vi "AddRealMeasure.vi"(6 "MeasureExecutionStatus (NOT_COMPLETED)":T1=enum."NOT_COMPLETED", 7 "MeasureTime (Now)":timestamp, 8 "error in":errorcluster, 9 "Precision (6)":u8=6, 10 "Value":dbl, 11 "StepRun in":refnum<class "StepRun.lvclass">) -> (0 "error out":errorcluster, 2 "RealMeasure":refnum<class "RealMeasure.lvclass">, 3 "StepRun out":refnum<class "StepRun.lvclass">)   [LabVIEW 2021, in "ProligentXMLGenerator.lvlib" / "StepRun.lvclass"]
doc: "Add a Measure.\n\nDefines the value acquired by the measure.\nMeasures are globaly unique by their MeasureId property."
uses:
  StepRun.lvclass
  StepRun.lvclass/StepRun.ctl
  Measure/RealMeasure/RealMeasure.lvclass
  C:/Projects/proligent-xml-generator-labview/src/ProligentXMLGenerator/Measure/Measure/Measure.lvclass
  C:/Projects/proligent-xml-generator-labview/src/ProligentXMLGenerator/Measure/RealMeasure/RealMeasure.lvclass
  Base/ExecutionStatus/Value.ctl
  Base/ExecutionStatus/ExecutionStatus.lvclass
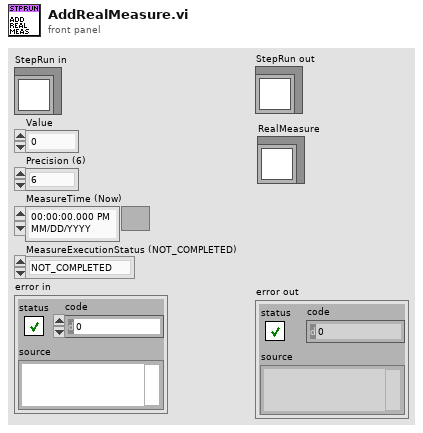
[diagram p1: front panel]
types:
  T1 = typedef "ProligentXMLGenerator.lvlib/ExecutionStatus.lvclass/Value.ctl" = enum16{"PASS", "FAIL", "NOT_COMPLETED", "ABORTED"}
  T2 = typedef "ProligentXMLGenerator.lvlib/StepRun.lvclass/Data.ctl" = cluster{"Name":string, "Measures":refnum<class "Measure.lvclass">[], "FailureReferences":refnum<class "FailureReference.lvclass">[], "Characteristics":refnum<class "Characteristic.lvclass">[], "Documents":refnum<class "Document.lvclass">[], "CustomData":refnum<class "CustomData.lvclass">, "StepExecutionStatus":refnum<class "ExecutionStatus.lvclass">, "StepRunId":refnum<class "Guid.lvclass">, "StepName":refnum<class "NonEmptyString_255.lvclass">, "StartDate":refnum<class "DateTime.lvclass">, "EndDate":refnum<class "DateTime.lvclass">, "TimeZoneInfoId":string}
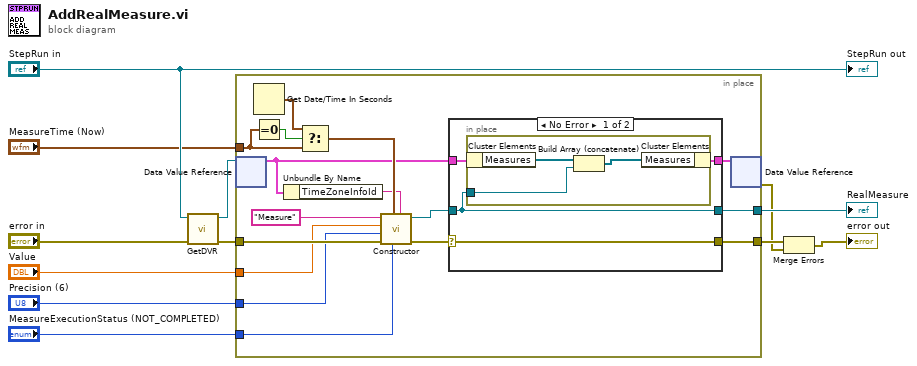
[diagram p0: block diagram]
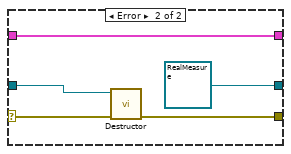
[diagram p2: hidden frame]
diagram:
  n1 = call "GetDVR.vi"("error in"="error in", "StepRun"="StepRun in") -> ("error out"=w5:errorcluster, "DVRReference"=w4:refnum<data-value>)  [unwired: 8 in]
  n2 = in-place "In Place Element Structure" {
    in-place-border: "Value" -> [w21]
    in-place-border: [w28] -> w6
    in-place-border: w5 -> [w22]
    in-place-border: [w26] -> w8
    in-place-border: "Precision (6)" -> [w19]
    in-place-border: "MeasureExecutionStatus (NOT_COMPLETED)" -> [w20]
    in-place-border: "MeasureTime (Now)" -> [w18]
    n3 = in-place-dvr #1(w4) -> (w14:T2)  [unwired: 1 out]
    n4 = Get Date/Time In Seconds() -> (seconds since 1Jan1904=w16:timestamp)
    n5 = Equal To 0?(x=w18) -> (x = 0?=w17:bool)
    n6 = Unbundle By Name(w14) -> ("TimeZoneInfoId"=w13:string)
    n7 = Select(t=w16, s=w17, f=w18) -> (s? t:f=w15:timestamp)
    n8 = call "Constructor.vi"("TimeZoneInfoId"=w13, "MeasureExecutionStatus"=w20, "MeasureTime"=w15, "error in"=w22, "Precision (6)"=w19, "Value"=w21, "Name"="Measure") -> ("error out"=w24:errorcluster, "RealMeasure"=w25:refnum<class "RealMeasure.lvclass">)  [unwired: 3 in]
    n9 = case shown="No Error" w24 {
      selector: w24 -> [w32 w39]
      tunnel: [w29 w40] -> w27
      tunnel: [w32 w38] -> w28
      tunnel: w25 -> [w31 w37]
      tunnel: w14 -> [w30 w40]
      tunnel: [w31 refnum<class "RealMeasure.lvclass"> refnum ("ProligentResultProcessor:RealMeasure")] -> w26
      frame No Error {
        n10 = in-place "In Place Element Structure" {
          in-place-border: w31 -> [w35]
          n11 = in-place-cluster #2(w30) -> ("Measures"=w34:refnum<class "Measure.lvclass">[])
          n12 = Build Array (concatenate)(w34, w35) -> (w33:refnum<class "Measure.lvclass">[])
          n13 = in-place-cluster #2("Measures"=w33) -> (w29:T2)
        }
      }
      frame Error {
        n14 = call "Destructor.vi"("error in"=w39, "RealMeasure"=w37) -> ("error out"=w38:errorcluster)  [unwired: 9 in]
      }
    }
    n15 = in-place-dvr #1(w27) -> (w3:errorcluster)  [unwired: 1 out]
  }
  "RealMeasure" <- w8
  n16 = Merge Errors(w6, w3) -> (→"error out":errorcluster)
  "StepRun out" <- "StepRun in"
